vi "Auto Outtake.vi"(11 "outtakeSpeed":dbl) -> ()   [LabVIEW 2017]
uses:
  Common Code/Intake Mode.ctl
  Robot Global Data.vi
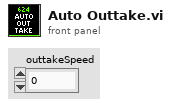
[diagram p1: front panel]
types:
  T1 = typedef "Intake Mode.ctl" = enum16{"Auto", "Semi Auto", "Manual"}
  T2 = typedef "Intake Command Cluster.ctl" = cluster{"Intake Mode":T1, "Intake States":T3, "Manual Roller Power":dbl, "Manual Close?":bool, "Manual Lift Power":dbl, "Override Lift?":bool, "Override Angle":dbl}
  T3 = typedef "Intake States.ctl" = enum16{"Curl Up", "Override Angle", "Idle", "Drop Mid", "Drop Low", "Outtake", "Intake"}
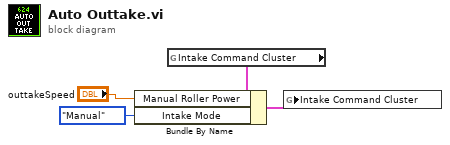
[diagram p0: block diagram]
diagram:
  n1 = global read "Robot Global Data.vi" "Intake Command Cluster"() -> (w4:T2)
  n2 = Bundle By Name(cluster=w4, "Manual Roller Power"="outtakeSpeed", "Intake Mode"=Intake_Mode."Manual") -> (w3:T2)
  n3 = global write "Robot Global Data.vi" "Intake Command Cluster"(w3) -> ()
